vi "updateIntegrationTime.vi"(8 "error in (no error)":errorcluster, 9 "InternalCommandId.lvclass":refnum<class "InternalCommandId.lvclass">, 10 "intTime":sgl, 11 "ElectrometerController in":refnum<class "ElectrometerController.lvclass">) -> (0 "error out":errorcluster, 3 "ElectrometerController out":refnum<class "ElectrometerController.lvclass">)   [LabVIEW 2016, in "ElectrometerController.lvclass"]
uses:
  ElectrometerController.lvclass
  Electrometer/State/ElectrometerState.lvclass
  InternalCommandId/InternalCommandId.lvclass
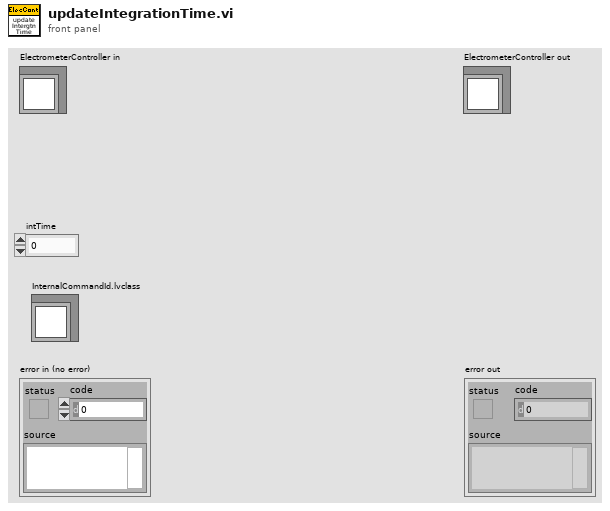
[diagram p1: front panel]
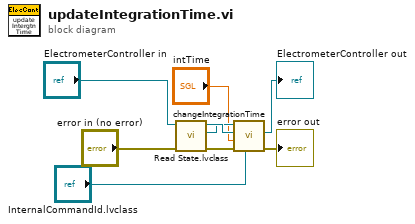
[diagram p0: block diagram]
diagram:
  n1 = call-dynamic "Read State.lvclass.vi"("error in (no error)"="error in (no error)", "ElectrometerController in"="ElectrometerController in") -> ("error out"=w7:errorcluster, "ElectrometerState"=w8:refnum<class "ElectrometerState.lvclass">, "ElectrometerController out"=w9:refnum<class "ElectrometerController.lvclass">)  [unwired: 7 in]
  n2 = call-dynamic "changeIntegrationTime.vi"("InternalCommandId.lvclass"="InternalCommandId.lvclass", "error in (no error)"=w7, "IntegrationTime"="intTime", "ElectrometerController in"=w9, "ElectrometerState in"=w8) -> ("error out"=→"error out":errorcluster, "ElectrometerController out"=→"ElectrometerController out":refnum<class "ElectrometerController.lvclass">)  [unwired: 4 in, 1 out]
